vi "Generic Prompt.vi"() -> ()   [LabVIEW 2014]
uses:
  Controls/Instrument ID Object.ctl
  SetUp VIs/Instrument Finder/Instrument Finder.lvclass
  Subpanel Inserter Messages/Insert Into Subpanel Msg/Insert Into Subpanel Msg.lvclass/Insert Into Subpanel Msg.ctl
  <vilib>/ActorFramework/Message Enqueuer/Message Enqueuer.lvclass/Message Enqueuer.ctl
  <vilib>/ActorFramework/Message Enqueuer/Enqueue.vi
  <vilib>/ActorFramework/Message Priority Queue/Priority Enqueue.vi
  Subpanel Inserter Messages/Insert Into Subpanel Msg/Insert Into Subpanel Msg.lvclass
  <vilib>/ActorFramework/Stop Msg/Stop Msg.lvclass
  <vilib>/ActorFramework/Actor/Actor.lvclass
panel:
  out "error out":errorcluster
  out "List of Instruments Out":T1[](array[typedef])
  in  "Stop Button":bool
  in  "Previous Button":bool
  in  "Next Button":bool
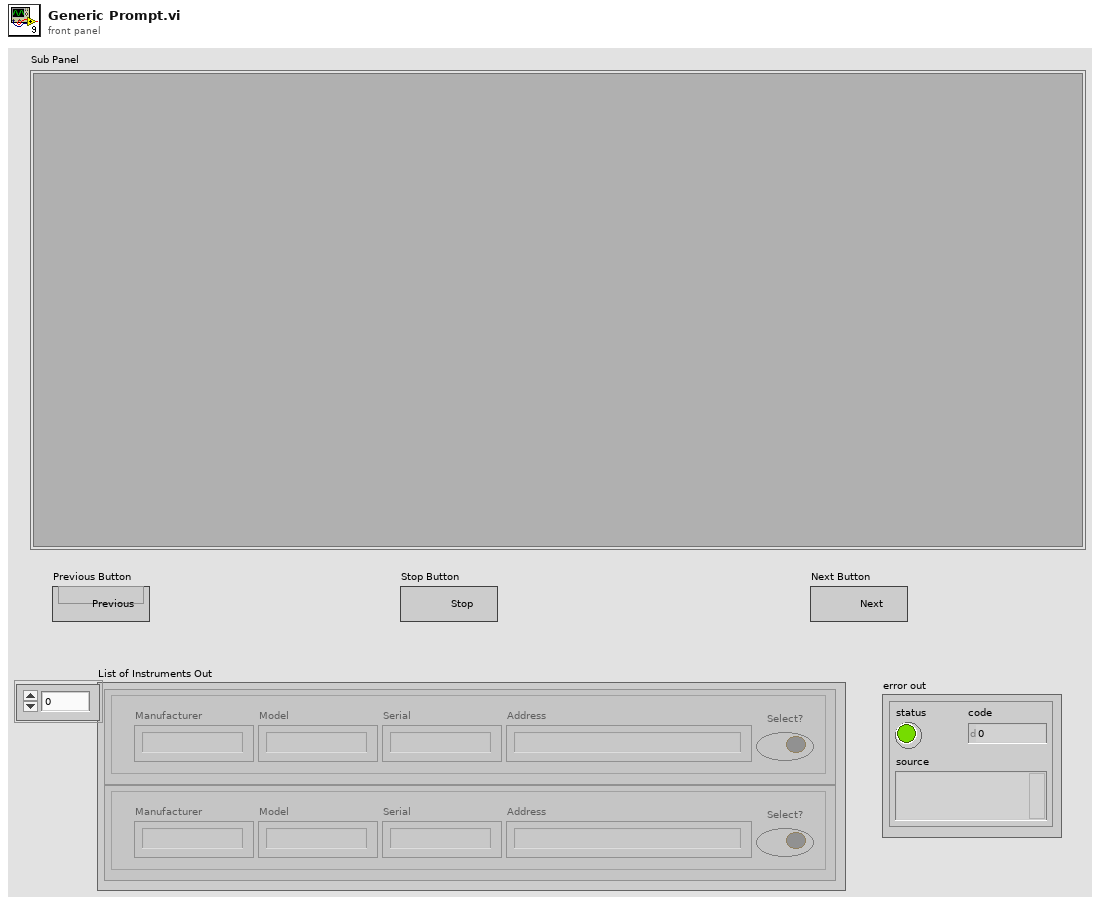
[diagram p1: front panel]
types:
  T1 = typedef "Instrument ID Object.ctl" = cluster{"Manufacturer":string, "Model":string, "Serial":string, "Address":string, "Select?":bool}
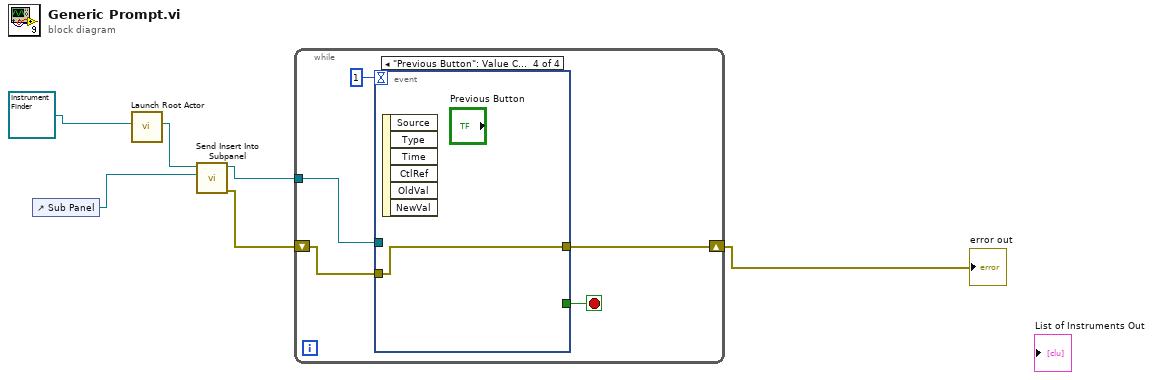
[diagram p0: block diagram]
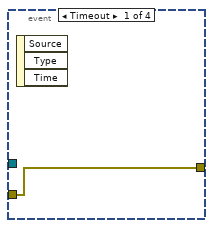
[diagram p2: hidden frame]
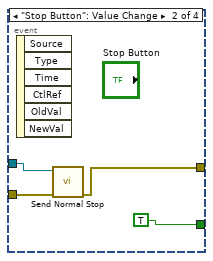
[diagram p3: hidden frame]
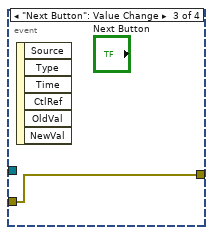
[diagram p4: hidden frame]
diagram:
  n1 = control-ref of="Sub Panel"() -> (w6:refnum<vi>)
  n2 = call <vilib>:"Launch Root Actor.vi"("Actor"=refnum<class "Instrument Finder.lvclass"> refnum ("SetUp VIs.lvlib:Instrument Finder.lvclass")) -> ("Actor's Enqueuer"=w4:refnum<class "Message Enqueuer.lvclass">)  [unwired: 9 in, 1 out]
  n3 = call "Send Insert Into Subpanel.vi"("SubPanel Ref"=w6, "Message Enqueuer"=w4) -> ("error out"=w2:errorcluster, "Message Enqueuer out"=w3:refnum<class "Message Enqueuer.lvclass">)  [unwired: 8 in]
  n4 = while {
    tunnel: w3 -> [w10]
    shift-right: [w7] -> w1
    shift-left: w2 -> [w8]
    stop <- w9 stop-if-true
    n5 = event shown="[3] \"Previous Button\": Value Change" {
      selector: _ -> [_ _ _ _]
      dyn-events: _ -> [_ _ _ _]
      timeout: 1 -> [_ _ _ _]
      tunnel: w10 -> [_ w15 _ _]
      tunnel: [_ TRUE _ _] -> w9
      tunnel: w8 -> [w12 w14 w17 w18]
      tunnel: [w12 w13 w17 w18] -> w7
      event Timeout {
        n6 = event-data() -> ()  [unwired: 1 in, 3 out]
      }
      event "Stop Button": Value Change {
        n7 = event-data() -> ()  [unwired: 1 in, 6 out]
        n8 = call <vilib>:"Send Normal Stop.vi"("error in (no error)"=w14, "Message Enqueuer"=w15) -> ("error out"=w13:errorcluster)  [unwired: 9 in]
      }
      event "Next Button": Value Change {
        n9 = event-data() -> ()  [unwired: 1 in, 6 out]
      }
      event "Previous Button": Value Change {
        n10 = event-data() -> ()  [unwired: 1 in, 6 out]
      }
    }
  }
  "error out" <- w1
